vi "EvEstMqEst.vi"() -> ()   [LabVIEW 2020]
uses:
  idle.ctl
panel:
  in  "Reject Coins":bool
  in  "Cancel":bool
  in  "Selected":bool
  in  "Enough Coins":bool
  in  "Coin Inserted":bool
  out "Enum":T1
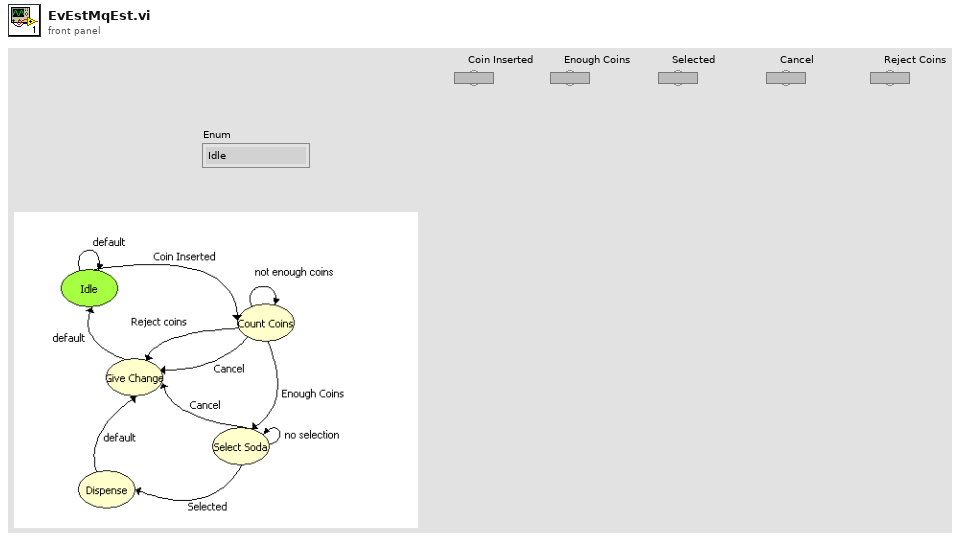
[diagram p1: front panel]
types:
  T1 = typedef "idle.ctl" = enum16{"Idle", "Count Coins", "Give Change", "Select Soda", "Dispense"}
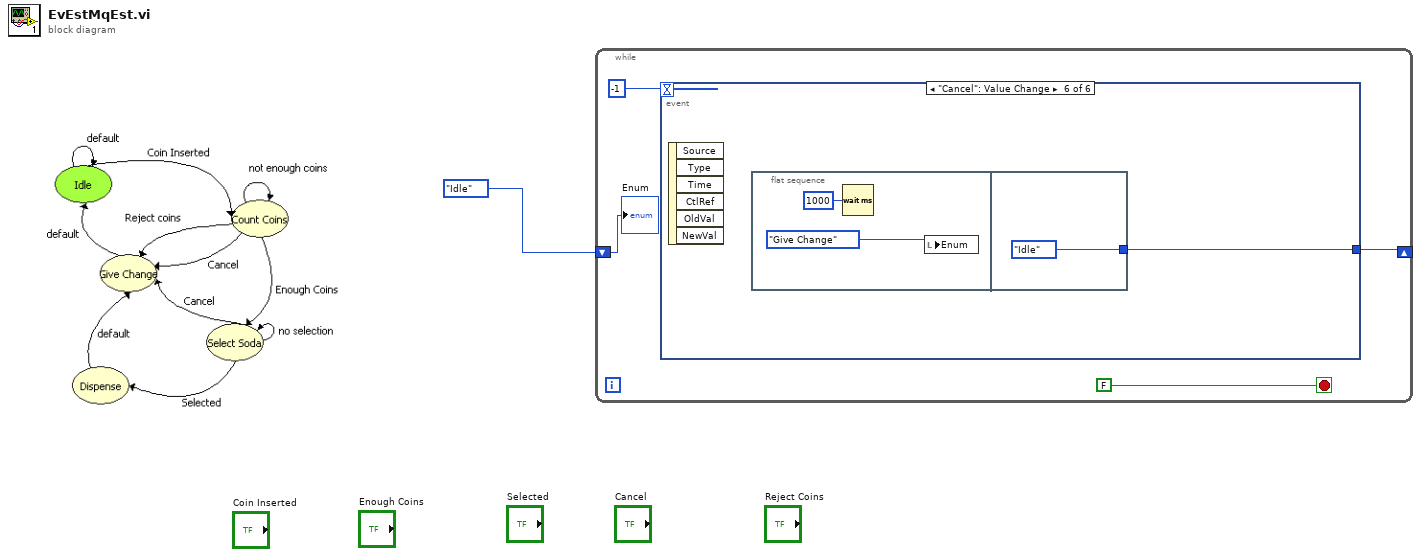
[diagram p0: block diagram]
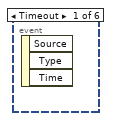
[diagram p2: hidden frame]
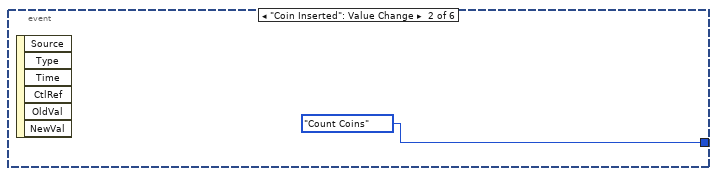
[diagram p3: hidden frame]
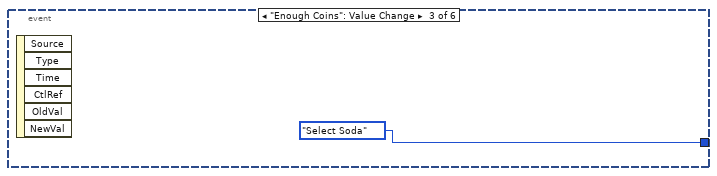
[diagram p4: hidden frame]
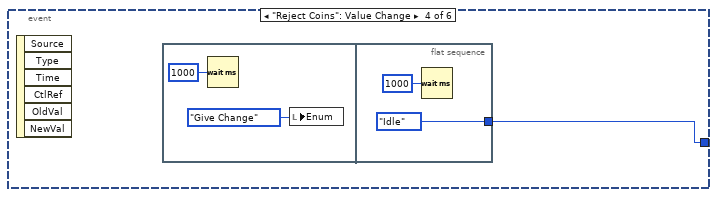
[diagram p5: hidden frame]
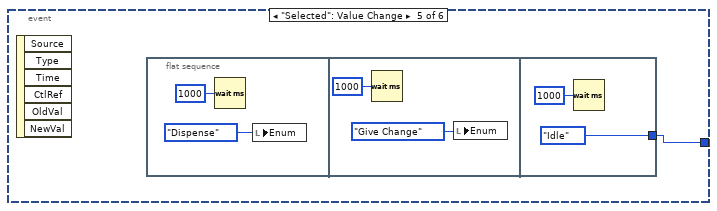
[diagram p6: hidden frame]
diagram:
  n1 = while {
    shift-right: [w2] -> _
    shift-left: idle."Idle" ("Enum") -> [w3]
    stop <- FALSE stop-if-true
    n2 = event shown="[5] \"Cancel\": Value Change" {
      selector: _ -> [_ _ _ _ _ _]
      dyn-events: _ -> [_ _ _ _ _ _]
      timeout: -1 -> [_ _ _ _ _ _]
      tunnel: [_ idle."Count Coins" ("Enum") idle."Select Soda" ("Enum") w8 w13 w20] -> w2
      event Timeout {
        n3 = event-data() -> ()  [unwired: 1 in, 3 out]
      }
      event "Coin Inserted": Value Change {
        n4 = event-data() -> ()  [unwired: 1 in, 6 out]
      }
      event "Enough Coins": Value Change {
        n5 = event-data() -> ()  [unwired: 1 in, 6 out]
      }
      event "Reject Coins": Value Change {
        n6 = event-data() -> ()  [unwired: 1 in, 6 out]
        n7 = flat-sequence {
          tunnel: [idle."Idle" ("Enum")] -> w8
          frame #0 {
            n8 = Wait (ms)(milliseconds to wait=u32 1000) -> ()  [unwired: 1 out]
            n9 = local write "Enum"(idle."Give Change" ("Enum")) -> ()
          }
          frame #1 {
            n10 = Wait (ms)(milliseconds to wait=u32 1000) -> ()  [unwired: 1 out]
          }
        }
      }
      event "Selected": Value Change {
        n11 = event-data() -> ()  [unwired: 1 in, 6 out]
        n12 = flat-sequence {
          tunnel: [idle."Idle" ("Enum")] -> w13
          frame #0 {
            n13 = Wait (ms)(milliseconds to wait=u32 1000) -> ()  [unwired: 1 out]
            n14 = local write "Enum"(idle."Dispense" ("Enum")) -> ()
          }
          frame #1 {
            n15 = Wait (ms)(milliseconds to wait=u32 1000) -> ()  [unwired: 1 out]
            n16 = local write "Enum"(idle."Give Change" ("Enum")) -> ()
          }
          frame #2 {
            n17 = Wait (ms)(milliseconds to wait=u32 1000) -> ()  [unwired: 1 out]
          }
        }
      }
      event "Cancel": Value Change {
        n18 = event-data() -> ()  [unwired: 1 in, 6 out]
        n19 = flat-sequence {
          tunnel: [idle."Idle" ("Enum")] -> w20
          frame #0 {
            n20 = Wait (ms)(milliseconds to wait=u32 1000) -> ()  [unwired: 1 out]
            n21 = local write "Enum"(idle."Give Change" ("Enum")) -> ()
          }
          frame #1 {
          }
        }
      }
    }
    "Enum" <- w3
  }
